vi "registerPublisherReply.vi"(1 "Response":string="HTTP/1.0 200 OK\r\nServer: BaseHTTP/0.3 Python/2.7.1\r\nDate: Fri, 24 May 2013 07:09:25 GMT\r\nContent-type: text/xml\r\nContent-length: 296\r\n\r\n<?xml version='1.0'?>\n<methodResponse>\n<params>\n<param>\n<value><array><data>\n<value><int>1</int></value>\n<value><string>Unregistered [/labview] as provider of [/robot/head/command_head_nod]</string></value>\n<value><int>1</int></value>\n</data></array></value>\n</param>\n</params>\n</methodResponse>\n") -> (0 "Response":T1)   [LabVIEW 2012]
doc: "Takes XML from a register publisher request and returns a cluster with \n-Code\n-Status Message\n-arrary of APIs"
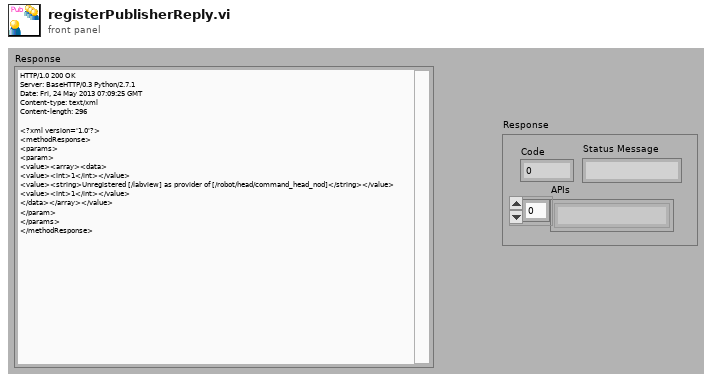
[diagram p1: front panel]
types:
  T1 = cluster{"Code":i32, "Status Message":string, "APIs":string[]}
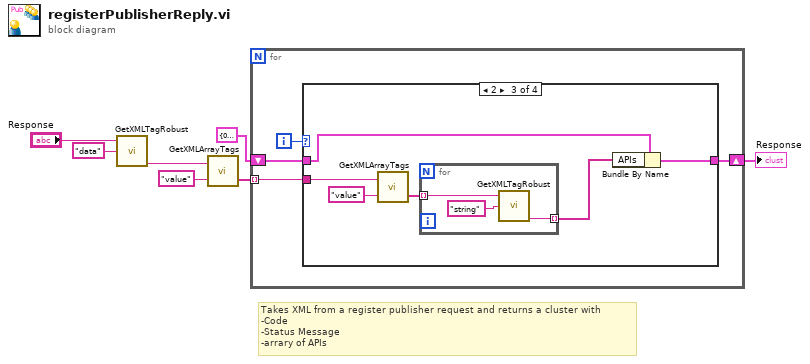
[diagram p0: block diagram]
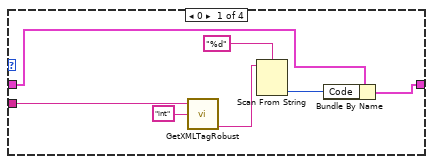
[diagram p2: hidden frame]
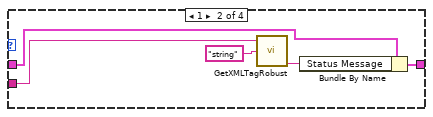
[diagram p3: hidden frame]
diagram:
  # "Takes XML from a register publisher request and returns a cluster with \n-Code\n-Status Message\n-arrary of APIs"
  n1 = call "GetXMLTagRobust.vi"("Tag"="data", "String"="Response") -> ("value"=w5:string)  [unwired: 1 in, 3 out]
  n2 = call "GetXMLArrayTags.vi"("ArrayTag"="value", "String"=w5) -> ("Array"=w3:string[])  [unwired: 1 out]
  n3 = for {
    tunnel: w3 -> [w9] mode=indexing
    shift-right: [w8] -> w1
    shift-left: T1 {"Code"=0, "Status Message"="", "APIs"=[]} ("Response") -> [w10]
    i -> [w11]
    n4 = case shown="2" w11 {
      tunnel: w10 -> [w13 w21 w26 w33]
      tunnel: w9 -> [w18 w23 w29 _]
      tunnel: [w12 w20 w25 w33] -> w8
      frame 0 {
        n5 = call "GetXMLTagRobust.vi"("Tag"="int", "String"=w18) -> ("value"=w15:string)  [unwired: 1 in, 3 out]
        n6 = Scan From String(format string="%d", input string=w15) -> (output 1=w14:i32)  [unwired: 3 in, 3 out]
        n7 = Bundle By Name(cluster=w13, "Code"=w14) -> (w12:T1)
      }
      frame 1 {
        n8 = call "GetXMLTagRobust.vi"("Tag"="string", "String"=w23) -> ("value"=w19:string)  [unwired: 1 in, 3 out]
        n9 = Bundle By Name(cluster=w21, "Status Message"=w19) -> (w20:T1)
      }
      frame 2 {
        n10 = call "GetXMLArrayTags.vi"("ArrayTag"="value", "String"=w29) -> ("Array"=w27:string[])  [unwired: 1 out]
        n11 = for {
          tunnel: w27 -> [w32] mode=indexing
          tunnel: [w30] -> w24 mode=indexing
          n12 = call "GetXMLTagRobust.vi"("Tag"="string", "String"=w32) -> ("value"=w30:string)  [unwired: 1 in, 3 out]
        }
        n13 = Bundle By Name(cluster=w26, "APIs"=w24) -> (w25:T1)
      }
      frame Default {
      }
    }
  }
  "Response" <- w1
